vi "WPI_CameraOpenAndSetVideoMode.vi"(8 "error in (no error)":errorcluster, 9 "USB JPEG":bool, 11 "Camera Address":string) -> (0 "error out":errorcluster)   [LabVIEW 2017]
uses:
  <vilib>/vision/driver/NI_Vision_Acquisition_Software.lvlib
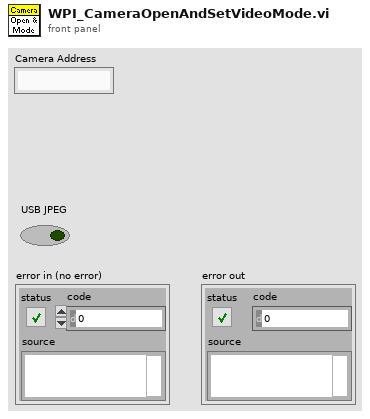
[diagram p1: front panel]
types:
  T1 = cluster{"Video Mode":u32, "Video Mode Name":string}[]
  T2 = typedef "IMAQdx.ctl" = refnum<k21>
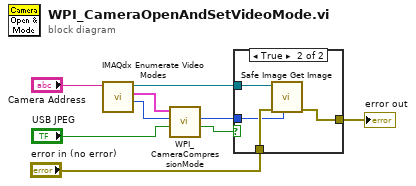
[diagram p0: block diagram]
diagram:
  n1 = call <vilib>:"IMAQdx Enumerate Video Modes.vi"("Session In"="Camera Address") -> ("Current Mode"=w7:u32, "Video Modes"=w8:T1, "Session Out"=w6:T2)  [unwired: 7 in, 1 out]
  n2 = call <vilib>:"WPI_CameraCompressionMode.vi"("JPEG"="USB JPEG", "VM Index"=w7, "Video Modes"=w8) -> ("Changed"=w5:bool, "VM Index out"=w4:i32)  [unwired: 7 in]
  n3 = case shown="True" w5 {
    tunnel: w4 -> [_ w11]
    tunnel: w6 -> [_ w12]
    tunnel: "error in (no error)" -> [w10 w13]
    tunnel: [w10 w14] -> w1
    frame False {
    }
    frame True {
      n4 = call <vilib>:"Safe Image Get Image.vi"("Video Mode"=w11, "error in"=w13, "Session In"=w12) -> ("error out"=w14:errorcluster)  [unwired: 5 in, 3 out]
    }
  }
  "error out" <- w1
